vi "Initialize.vi"(0 "VISA resource name":refnum<visa-resource-name>, 5 "ID Query? (T: Yes)":bool=TRUE, 7 "Reset? (T: Yes)":bool=TRUE, 11 "error in (no error)":errorcluster {"code" format="%.0x"}) -> (4 "VISA resource name out":refnum<visa-resource-name>, 15 "error out":errorcluster {"code" format="%.0x"})   [LabVIEW 2017, in "Agilent N6700 Series.lvlib"]
doc: "This VI passes the addressing information in the instrument decriptor to the Instr Open VI and returns the instrument ID. You can optionally reset the instrument by setting the front panel reset control. You must run this VI before using any of the instrument driver VIs for this instrument.\n\n<b>Notes:</b>\n\n(1) This instrument driver supports serial communication. If problems are encountered when using serial communication, it is recommended to try using baud rates less than 19,200 and hardware handshaking. \n\n(2) If you do wish to use the serial interface, set the serial settings on the instrument to be the same as the serial settings on the block diagram and in Measurement & Automation Explorer."
uses:
  Agilent N6700 Series.lvlib
panel:
  # "(c) 2004-2015  National Instruments.  ALL RIGHTS RESERVED."
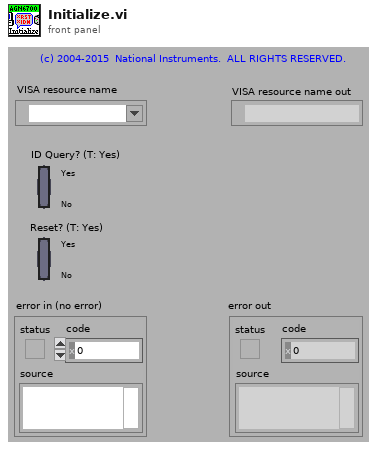
[diagram p1: front panel]
types:
  T1 = cluster{"Status":bool, "Code":i32, "Source (VI Name)":string}
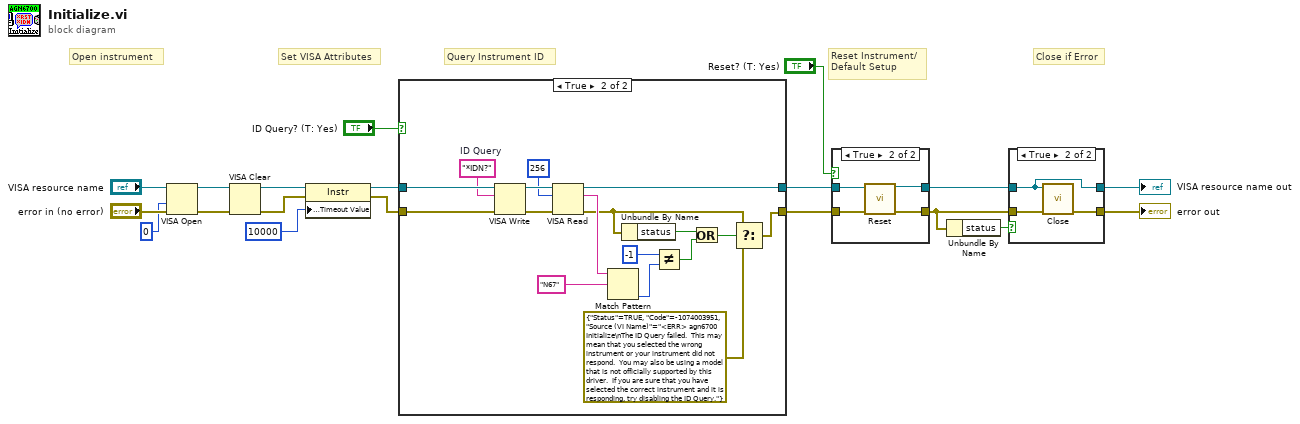
[diagram p0: block diagram]
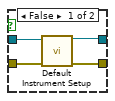
[diagram p3: hidden frame]
diagram:
  # "Set VISA Attributes"
  # "Close if Error"
  # "Query Instrument ID"
  # "Reset Instrument/\nDefault Setup"
  # "Open instrument"
  n1 = VISA Open(access mode=u32 0, error in (no error)="error in (no error)", VISA resource name="VISA resource name") -> (VISA resource name=w6:refnum<visa-resource-name>, error out=w5:errorcluster)  [unwired: 2 in]
  n2 = VISA Clear(VISA resource name=w6, error in (no error)=w5) -> (VISA resource name out=w4:refnum<visa-resource-name>, error out=w3:errorcluster)
  n3 = property class="Instr"(reference=w4, error in=w3, "General Settings:Timeout Value"=u32 10000) -> (reference out=w9:refnum<visa-resource-name>, error out=w8:errorcluster)
  n4 = case shown="True" "ID Query? (T: Yes)" {
    tunnel: [w20 w38] -> w18
    tunnel: [w21 w35] -> w19
    tunnel: w9 -> [w21 w36]
    tunnel: w8 -> [w20 w37]
    frame False {
    }
    frame True {
      w23 = "*IDN?"  # ID Query
      n5 = VISA Write(VISA resource name=w36, write buffer=w23, error in (no error)=w37) -> (VISA resource name out=w32:refnum<visa-resource-name>, error out=w30:errorcluster)  [unwired: 1 out]
      n6 = VISA Read(VISA resource name=w32, byte count=u32 256, error in (no error)=w30) -> (VISA resource name out=w35:refnum<visa-resource-name>, read buffer=w33:string, error out=w31:errorcluster)  [unwired: 1 out]
      n7 = Match Pattern(string=w33, regular expression="N67") -> (offset past match=w25:i32)  [unwired: 1 in, 3 out]
      n8 = Unbundle By Name(w31) -> ("status"=w28:bool)
      n9 = Not Equal?(x=-1, y=w25) -> (x != y?=w34:bool)
      n10 = Or(x=w28, y=w34) -> (x .or. y?=w29:bool)
      n11 = Select(t=w31, s=w29, f=T1 {"Status"=TRUE, "Code"=-1074003951, "Source (VI Name)"="<ERR> agn6700 Initialize\nThe ID Query failed.  This may mean that you selected the wrong instrument or your instrument did not respond.  You may also be using a model that is not officially supported by this driver.  If you are sure that you have selected the correct instrument and it is responding, try disabling the ID Query."}) -> (s? t:f=w38:T1)
    }
  }
  n12 = case shown="True" "Reset? (T: Yes)" {
    tunnel: w18 -> [w41 w43]
    tunnel: [w40 w46] -> w2
    tunnel: w19 -> [w42 w44]
    tunnel: [w39 w45] -> w15
    frame False {
      n13 = call "Default Instrument Setup.vi"("VISA resource name"=w42, "error in (no error)"=w41) -> ("VISA resource name out"=w39:refnum<visa-resource-name>, "error out"=w40:errorcluster)  [unwired: 12 in]
    }
    frame True {
      n14 = call "Reset.vi"("VISA resource name"=w44, "error in (no error)"=w43) -> ("VISA resource name out"=w45:refnum<visa-resource-name>, "error out"=w46:errorcluster)  [unwired: 12 in]
    }
  }
  n15 = Unbundle By Name(w2) -> ("status"=w1:bool)
  n16 = case shown="True" w1 {
    tunnel: w15 -> [w48 w50]
    tunnel: [w48 w50] -> w14
    tunnel: [w47 w51] -> w13
    tunnel: w2 -> [w47 w49]
    frame False {
    }
    frame True {
      n17 = call "Close.vi"("VISA resource name"=w50, "error in (no error)"=w49) -> ("error out"=w51:errorcluster)  [unwired: 13 in]
    }
  }
  "VISA resource name out" <- w14
  "error out" <- w13
